vi "Serial.vi"(8 "error in (no error)":errorcluster, 9 "Clear Log":bool, 10 "write buffer":string="UA[3]\r\n", 11 "VISA resource name":refnum<visa-resource-name>="COM6") -> (0 "error out":errorcluster, 2 "read buffer":string)   [LabVIEW 2017]
uses:
  <vilib>/Instr/_visa.llb/VISA Configure Serial Port (Instr).vi
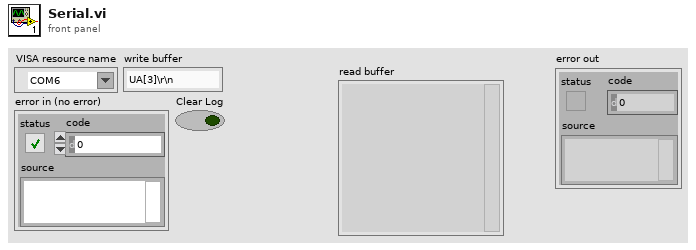
[diagram p1: front panel]
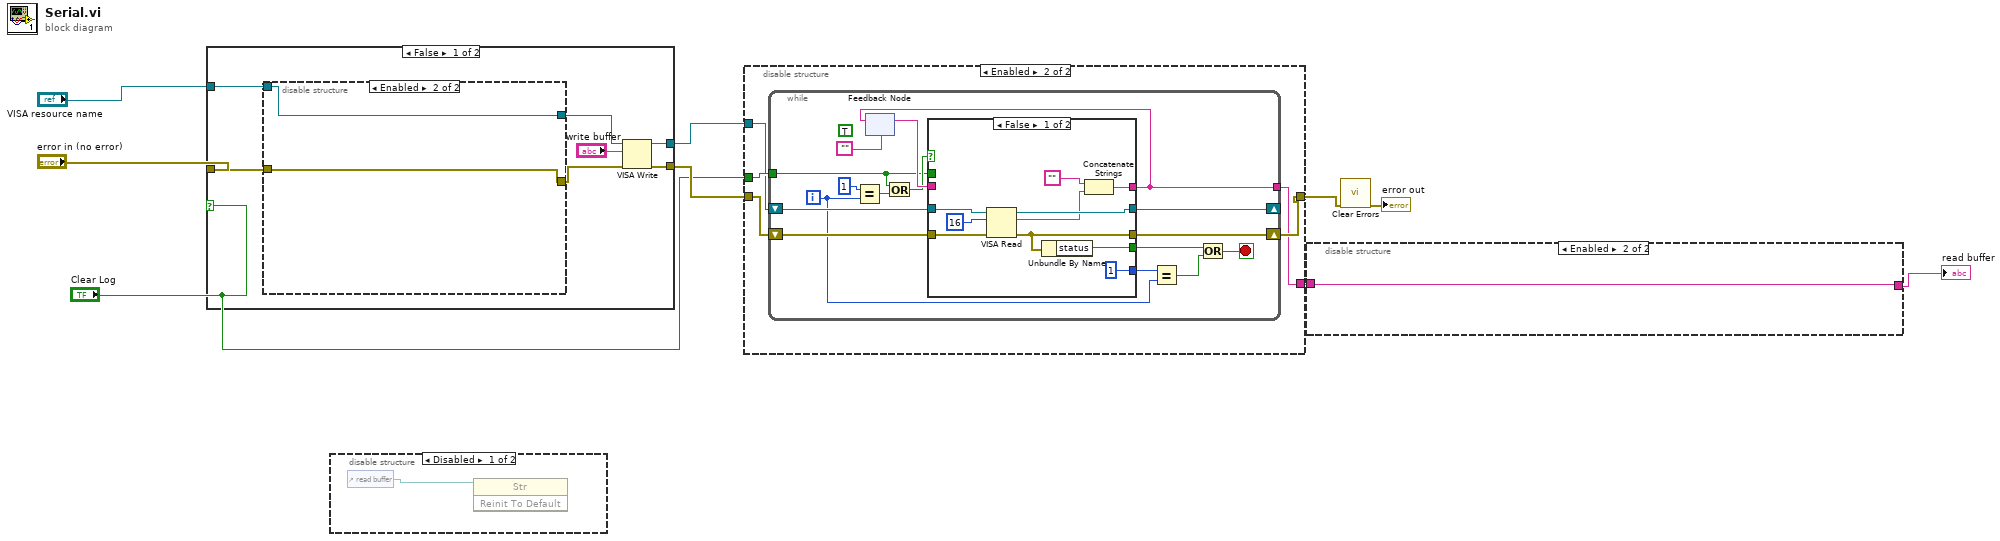
[diagram p0: block diagram]
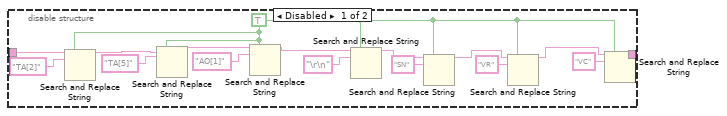
[diagram p2: hidden frame]
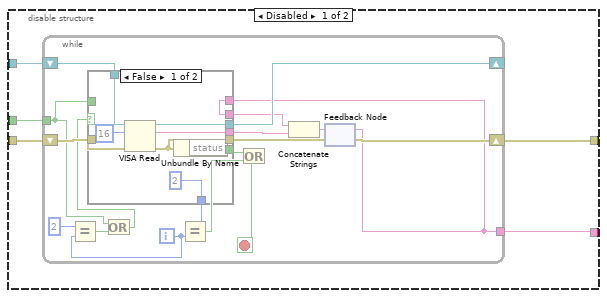
[diagram p3: hidden frame]
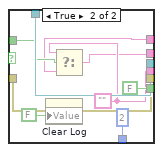
[diagram p4: hidden frame]
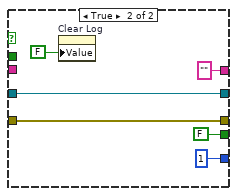
[diagram p5: hidden frame]
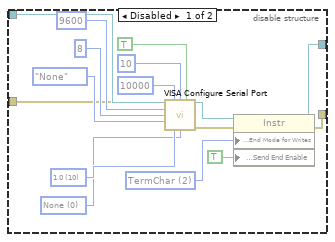
[diagram p7: hidden frame]
diagram:
  n1 = case shown="False" "Clear Log" {
    tunnel: "VISA resource name" -> [w11 w36]
    tunnel: "error in (no error)" -> [w10 w35]
    tunnel: [w14 w36] -> w5
    tunnel: [w13 w35] -> w4
    frame False {
      n2 = disable-structure shown="Enabled" {
        disable-tunnel: w11 -> [w32 w34]
        disable-tunnel: w10 -> [w26 w33]
        disable-tunnel: [w21 w34] -> w15
        disable-tunnel: [w20 w33] -> w16
        frame Disabled {
          w18 = u16 2 items=["None", "LastBit", "TermChar", "Break"] ("Serial Settings:Serial End Mode for Writes")
          w24 = u16 0 items=["None", "XON/XOFF", "RTS/CTS", "XON/XOFF & RTS/CTS", "DTR/DSR", "XON/XOFF & DTR/DSR"] ("flow control (0:none)")
          w25 = u16 10 items=["1.0"=10, "1.5"=15, "2.0"=20] ("stop bits (10: 1 bit)")
          n3 = call-poly "VISA Configure Serial Port"("VISA resource name"=w32, "timeout (10sec)"=u32 10000, "termination char\n(0xA = '\\n' = LF)"=u8 10 ("termination char\n(0xA = '\\n' = LF)"), "Enable Termination\nChar (T)"=TRUE ("Enable Termination\nChar (T)"), "baud rate (9600)"=u32 9600, "data bits (8)"=u16 8, "parity (0:none)"=enum16{"None", "Odd", "Even", "Mark", "Space"}."None", "error in (no error)"=w26, "stop bits (10: 1 bit)"=w25, "flow control (0:none)"=w24) -> ("VISA resource name out"=w22:refnum<visa-resource-name>, "error out"=w23:errorcluster)  [unwired: 4 in]
          n4 = property class="Instr"(reference=w22, error in=w23, "Serial Settings:End Mode for Writes"=w18, "Message Based Settings:Send End Enable"=TRUE) -> (reference out=w21:refnum<visa-resource-name>, error out=w20:errorcluster)
        }
        frame Enabled {
        }
      }
      n5 = VISA Write(VISA resource name=w15, write buffer="write buffer", error in (no error)=w16) -> (VISA resource name out=w14:refnum<visa-resource-name>, error out=w13:errorcluster)  [unwired: 1 out]
    }
    frame True {
    }
  }
  n6 = disable-structure shown="Disabled" {
    frame Disabled {
      n7 = control-ref of="read buffer"() -> (w37:refnum<vi>)
      n8 = invoke class="Str" method="Reinit To Default"(reference=w37) -> ()  [unwired: 2 in, 3 out]
    }
    frame Enabled {
    }
  }
  n9 = disable-structure shown="Enabled" {
    disable-tunnel: [w42 w79] -> w8
    disable-tunnel: w5 -> [w41 w81]
    disable-tunnel: w4 -> [w40 w80]
    disable-tunnel: "Clear Log" -> [w39 w82]
    disable-tunnel: [w38 w78] -> w2
    frame Disabled {
      n10 = while {
        shift-right: [w59] -> _
        shift-left: w41 -> [w53]
        shift-right: [w57] -> w42
        shift-left: w40 -> [w52]
        tunnel: [w50] -> w38
        tunnel: w39 -> [w43]
        i -> [w47]
        stop <- w55 stop-if-true
        n11 = Equal?(x=2, y=w47) -> (x = y?=w45:bool)
        n12 = Or(x=w43, y=w45) -> (x .or. y?=w44:bool)
        n13 = feedback #1() -> (w50:string)  [unwired: 1 in]
        n14 = case shown="False" w44 {
          tunnel: [w68 w77] -> w59
          tunnel: [w67 w71] -> w58
          tunnel: [w65 w76] -> w57
          tunnel: [w64 FALSE ("status")] -> w54
          tunnel: w53 -> [w63 w77]
          tunnel: w52 -> [w62 w76]
          tunnel: w50 -> [w61 w70]
          tunnel: [w61 w69] -> w49
          tunnel: [2 ("x") 2 ("x")] -> w48
          tunnel: w43 -> [_ w72]
          frame False {
            n15 = VISA Read(VISA resource name=w63, byte count=u32 16, error in (no error)=w62) -> (VISA resource name out=w68:refnum<visa-resource-name>, read buffer=w67:string, error out=w65:errorcluster)  [unwired: 1 out]
            n16 = Unbundle By Name(w65) -> ("status"=w64:bool)
          }
          frame True {
            w71 = ""
            n17 = property on="Clear Log" class="Bool (strict)"("Value"=FALSE ("Clear Log")) -> ()  [unwired: 2 in, 2 out]
            n18 = Select(t=w71, s=w72, f=w70) -> (s? t:f=w69:string)
          }
        }
        n19 = Equal?(x=w48, y=w47) -> (x = y?=w56:bool)
        n20 = Or(x=w54, y=w56) -> (x .or. y?=w55:bool)
        n21 = Concatenate Strings(w49, w58) -> (w51:string)
        n22 = feedback-in #1(w51) -> ()
      }
    }
    frame Enabled {
      n23 = while {
        shift-right: [w98] -> _
        shift-left: w81 -> [w95]
        shift-right: [w97] -> w79
        shift-left: w80 -> [w94]
        tunnel: w82 -> [w87]
        tunnel: [w83] -> w78
        i -> [w91]
        stop <- w84 stop-if-true
        (unwired) TRUE
        n24 = Equal?(x=1, y=w91) -> (x = y?=w89:bool)
        n25 = feedback #2("") -> (w93:string)
        n26 = Or(x=w87, y=w89) -> (x .or. y?=w88:bool)
        n27 = case shown="False" w88 {
          tunnel: [w108 w114] -> w98
          tunnel: [w106 w113] -> w97
          tunnel: [w105 FALSE ("status")] -> w96
          tunnel: w95 -> [w104 w114]
          tunnel: w94 -> [w103 w113]
          tunnel: w93 -> [_ _]
          tunnel: [1 ("x") 1 ("x")] -> w92
          tunnel: w87 -> [_ _]
          tunnel: [w101 ""] -> w83
          frame False {
            n28 = VISA Read(VISA resource name=w104, byte count=u32 16, error in (no error)=w103) -> (VISA resource name out=w108:refnum<visa-resource-name>, read buffer=w99:string, error out=w106:errorcluster)  [unwired: 1 out]
            n29 = Unbundle By Name(w106) -> ("status"=w105:bool)
            n30 = Concatenate Strings("", w99) -> (w101:string)
          }
          frame True {
            n31 = property on="Clear Log" class="Bool (strict)"("Value"=FALSE ("Clear Log")) -> ()  [unwired: 2 in, 2 out]
          }
        }
        n32 = feedback-in #2(w83) -> ()
        n33 = Equal?(x=w92, y=w91) -> (x = y?=w85:bool)
        n34 = Or(x=w96, y=w85) -> (x .or. y?=w84:bool)
      }
    }
  }
  n35 = disable-structure shown="Enabled" {
    disable-tunnel: w2 -> [w121 w131]
    disable-tunnel: [w116 w131] -> w1
    frame Disabled {
      w115 = TRUE ("replace all? (F)")
      n36 = Search and Replace String(replace all?=w115, input string=w121, search string="TA[2]" ("substring (\"\")")) -> (result string=w122:string)  [unwired: 5 in, 3 out]
      n37 = Search and Replace String(replace all?=w115, input string=w122, search string="TA[5]" ("substring (\"\")")) -> (result string=w128:string)  [unwired: 5 in, 3 out]
      n38 = Search and Replace String(replace all?=w115, input string=w128, search string="AO[1]" ("substring (\"\")")) -> (result string=w126:string)  [unwired: 5 in, 3 out]
      n39 = Search and Replace String(replace all?=w115, input string=w126, search string="\r\n" ("substring (\"\")")) -> (result string=w125:string)  [unwired: 5 in, 3 out]
      n40 = Search and Replace String(replace all?=w115, input string=w125, search string="SN") -> (result string=w119:string)  [unwired: 5 in, 3 out]
      n41 = Search and Replace String(replace all?=w115, input string=w119, search string="VR") -> (result string=w117:string)  [unwired: 5 in, 3 out]
      n42 = Search and Replace String(replace all?=w115, input string=w117, search string="VC") -> (result string=w116:string)  [unwired: 5 in, 3 out]
    }
    frame Enabled {
    }
  }
  "read buffer" <- w1
  n43 = call <vilib>:"Clear Errors.vi"("error in (no error)"=w8) -> ("error out"=→"error out":errorcluster)  [unwired: 5 in, 1 out]
